vi "Init.vi"(9 "Time":timestamp, 10 "Is Sync":bool) -> (3 "Base Sender out":refnum<class "Base Sender.lvclass">)   [LabVIEW 2020, in "jettl.lvlib" / "Sender.lvlib" / "Base Sender.lvclass"]
uses:
  Base Sender.lvclass
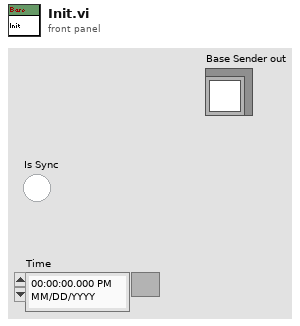
[diagram p1: front panel]
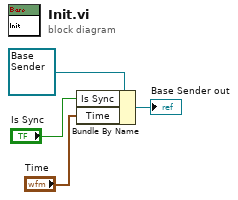
[diagram p0: block diagram]
diagram:
  n1 = Bundle By Name(cluster=refnum<class "Base Sender.lvclass"> refnum ("Base Sender out"), "Is Sync"="Is Sync", "Time"="Time") -> (→"Base Sender out":refnum<class "Base Sender.lvclass">)
